vi "Main.vi"() -> ()   [LabVIEW 2017]
doc: "This template is for the Queued Message Handler design pattern.\n\nThe Event Handling Loop generates messages based on user interface actions.\n\nThe Message Handling Loop processes messages generated by the Event Handling Loop, or by other messages. The messages are string values, so new messages can be added easily to the Message Cases case structure in the Message Handling Loop. Each message cluster can also provide an optional value for Message Data, which is a variant that can be converted to whatever message-specific data is required."
uses:
  Entry Display Data.ctl
  support/Message Queue/Enqueue Message (Single).vi
  <vilib>/Utility/error.llb/Error Cluster From Error Code.vi
  <vilib>/ErrorRing/Error Ring.xnode
  support/Message Queue/Message Queue.lvlib
  support/User Event - Stop/User Event - Stop.lvlib
panel:
  in  "Start":bool
  in  "Air Dry":bool
  in  "Tire Shine Foam":bool
  in  "Spot Free Rinse":bool
  in  "Low Pressure Wax":bool
  in  "High Pressure Wash":bool
  in  "Pre-Soak":bool
  in  "Bug Remover":bool
  in  "Under Body Wash":bool
  out "Display <Replace Me>":string
  in  "Do Something Else <Replace Me>":bool
  in  "Do Something <Replace Me>":bool
  in  "Exit":bool
  # "These controls have associated \"Value Changed\" events configured in the Event Structure on the diagram.\n\nReplace them (and reconfigure the Event Structure) with the controls you need for your application."
  # "This template is for the Queued Message Handler design pattern.\n\nSee the block diagram for more information on how to use this template."
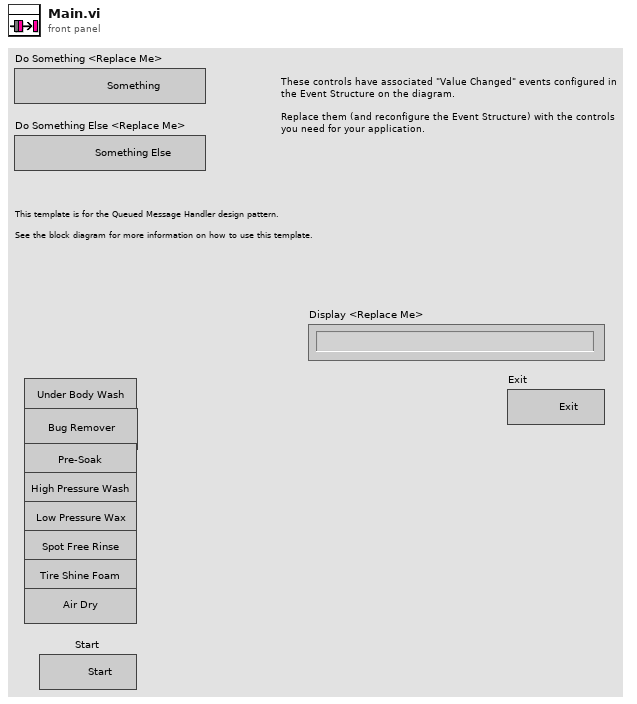
[diagram p1: front panel]
types:
  T1 = typedef "Entry Display Data.ctl" = cluster{"Under Body Wash":bool, "Bug Remover":bool, "Pre-soak":bool, " High Pressure Wash":bool, "Low Pressure  Wax":bool, "Spot Free Rinse":bool, " Tire Shine Foam":bool, " Air Dry":bool, "Vehicle Postion":bool}
  T2 = typedef "Message Queue.lvlib/All Message Queues.ctl" = cluster{"MHL":refnum<queue>, "Controller":refnum<queue>, "Display":refnum<queue>}
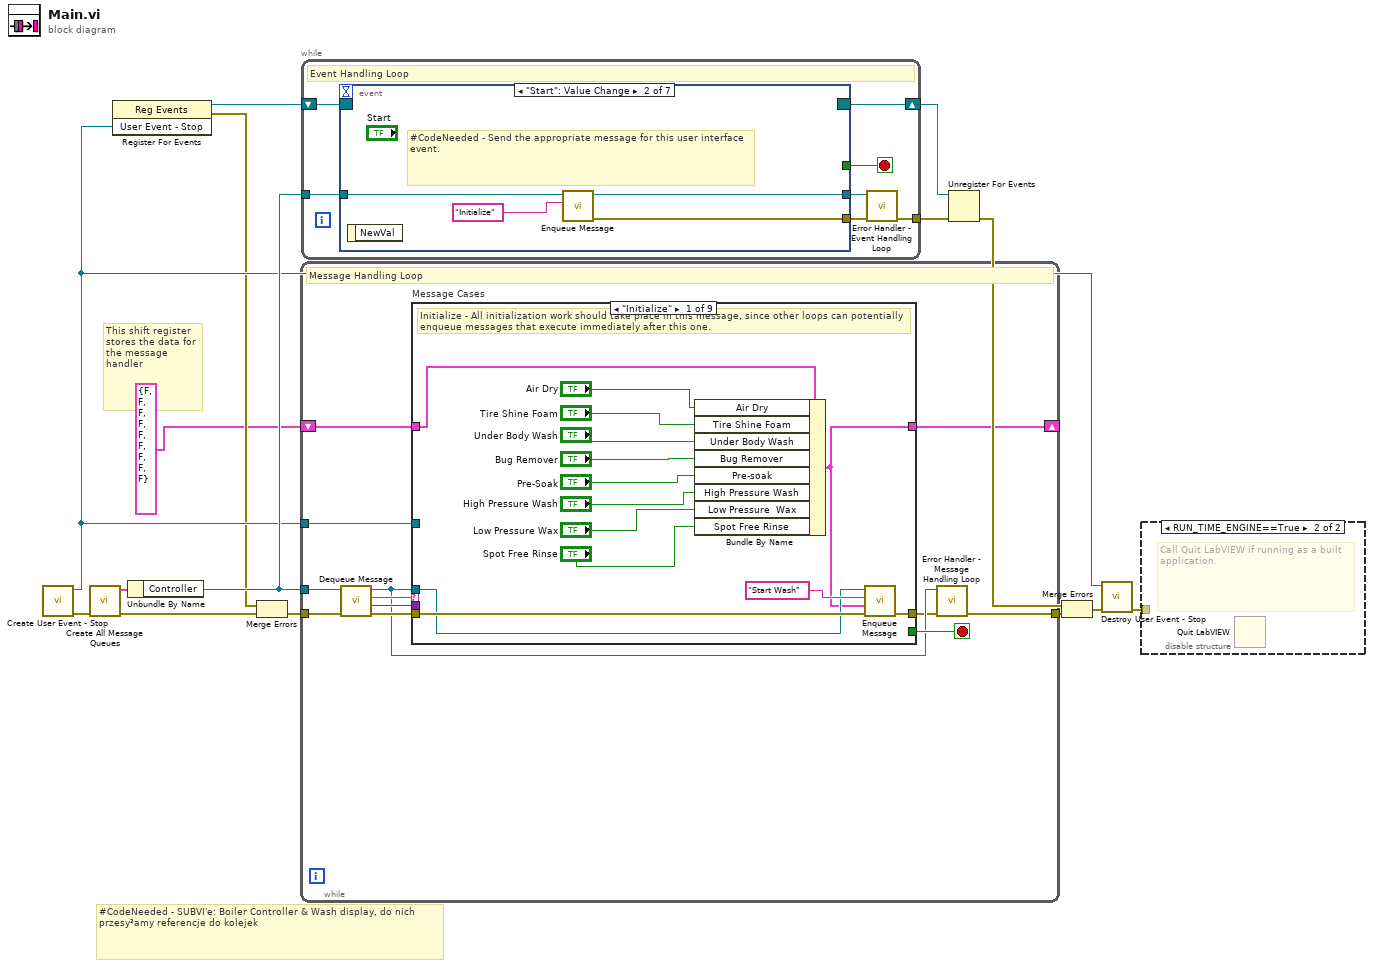
[diagram p0: block diagram]
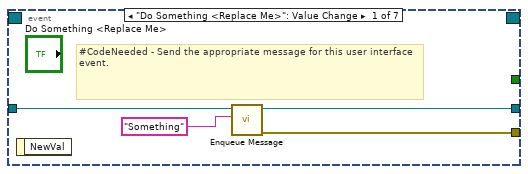
[diagram p3: hidden frame]
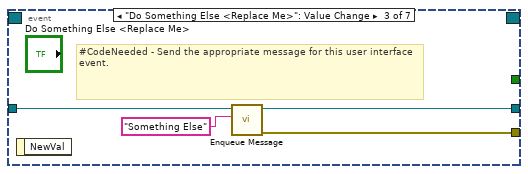
[diagram p4: hidden frame]
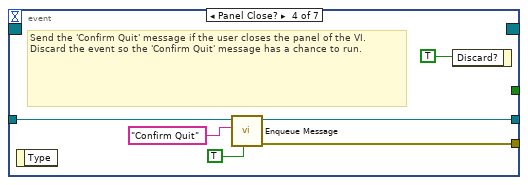
[diagram p5: hidden frame]
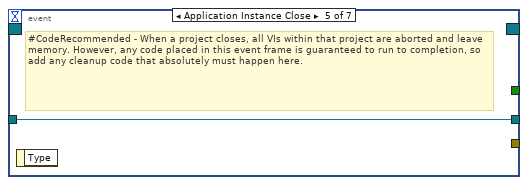
[diagram p6: hidden frame]
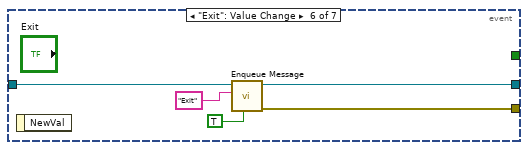
[diagram p7: hidden frame]
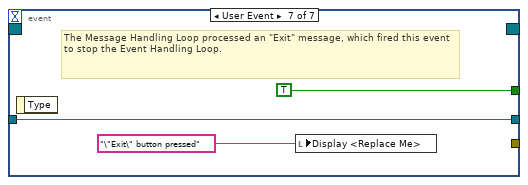
[diagram p8: hidden frame]
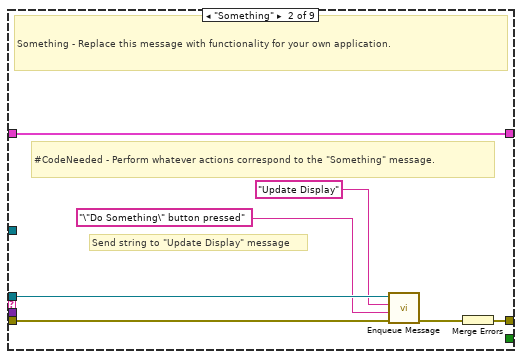
[diagram p9: hidden frame]
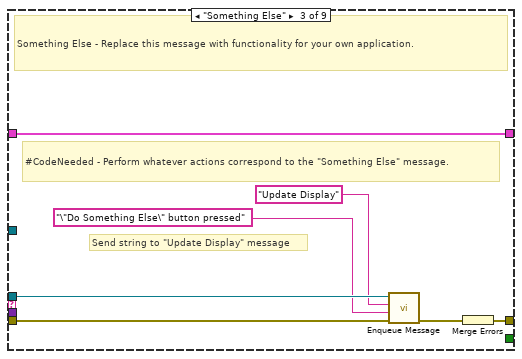
[diagram p10: hidden frame]
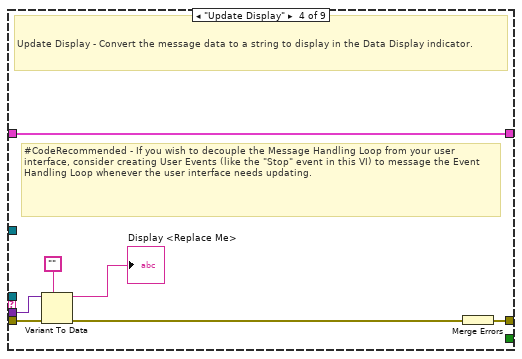
[diagram p11: hidden frame]
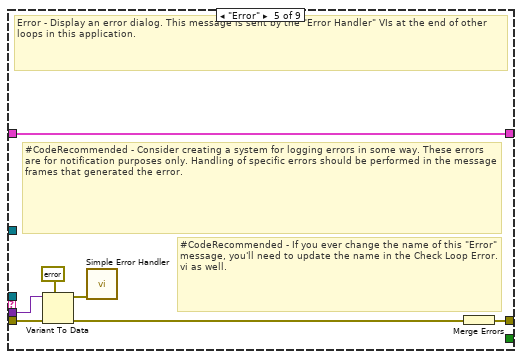
[diagram p12: hidden frame]
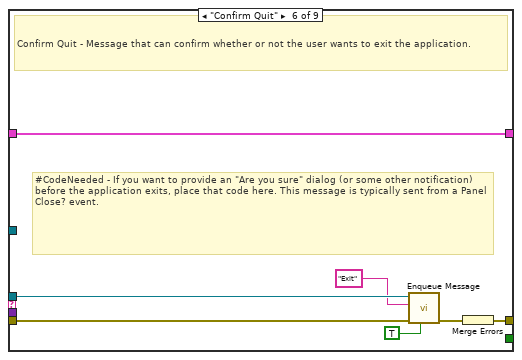
[diagram p13: hidden frame]
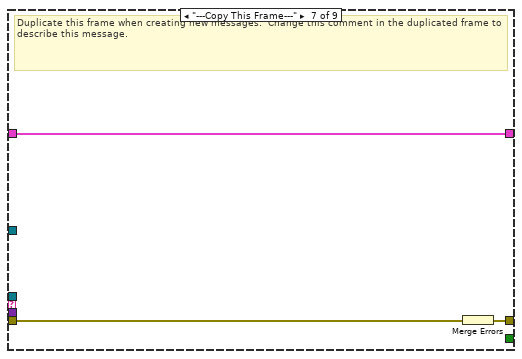
[diagram p14: hidden frame]
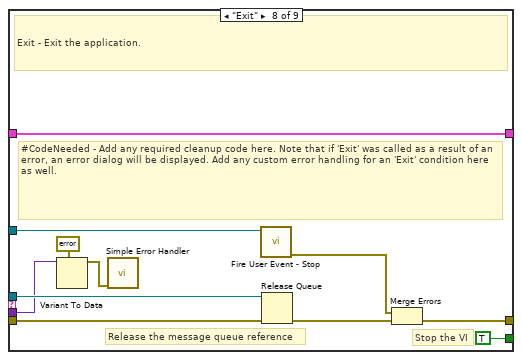
[diagram p15: hidden frame]
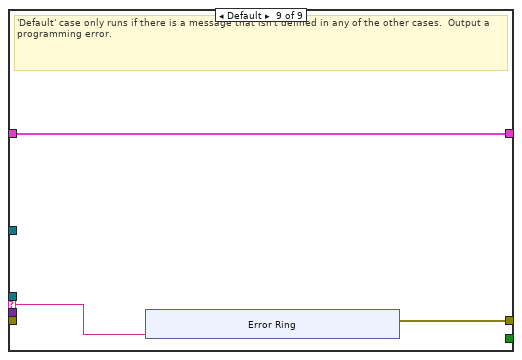
[diagram p16: hidden frame]
diagram:
  # "#CodeNeeded - SUBVI'e: Boiler Controller & Wash display, do nich przesy³amy referencje do kolejek"
  # "This shift register stores the data for the message handler"
  n1 = call "Create User Event - Stop.vi"() -> ("error out"=w11:errorcluster, "User Event - Stop"=w4:refnum<user-event>)  [unwired: 10 in]
  n2 = call "Create All Message Queues.vi"("error in (no error)"=w11) -> ("error out"=w15:errorcluster, "Message Queues out"=w14:T2)  [unwired: 9 in]
  n3 = register-events(w4) -> (reference out=w5:refnum<event-registration>, error out=w2:errorcluster)  [unwired: 2 in]
  n4 = Unbundle By Name(w14) -> ("Controller"=w12:refnum<queue>)
  n5 = Merge Errors(w2, w15) -> (w3:errorcluster)
  n6 = while {
    tunnel: w12 -> [w19]
    shift-right: [w26] -> _
    shift-left: T1 {"Under Body Wash"=FALSE, "Bug Remover"=FALSE, "Pre-soak"=FALSE, " High Pressure Wash"=FALSE, "Low Pressure  Wax"=FALSE, "Spot Free Rinse"=FALSE, " Tire Shine Foam"=FALSE, " Air Dry"=FALSE, "Vehicle Postion"=FALSE} ("Cluster") -> [w27]
    tunnel: w4 -> [w24]
    tunnel: w3 -> [w23]
    tunnel: [w17] -> w13
    stop <- w25 stop-if-true
    # "Message Handling Loop"
    n7 = call "Dequeue Message.vi"("error in (no error)"=w23, "Message Queue"=w19) -> ("error out"=w22:errorcluster, "Message Data"=w20:variant, "Message"=w21:string, "dup Message Queue"=w18:refnum<queue>)  [unwired: 6 in]
    n8 = case "Message Cases" shown="\"Initialize\"" w21 {
      selector: w21 -> [_ _ _ _ _ _ _ _ w91]
      tunnel: w18 -> [w38 w44 w51 _ _ w72 _ w90 _]
      tunnel: w22 -> [w40 w46 w53 w60 w69 w76 w79 w83 _]
      tunnel: [w41 w47 w54 w61 w63 w74 w77 w86 w92] -> w16
      tunnel: w27 -> [w29 w48 w55 w62 w68 w75 w78 w89 w93]
      tunnel: [w28 w48 w55 w62 w68 w75 w78 w89 w93] -> w26
      tunnel: [_ _ _ _ _ _ _ TRUE _] -> w25
      tunnel: w20 -> [_ _ _ w59 w67 _ _ w80 _]
      tunnel: w24 -> [_ _ _ _ _ _ _ w85 _]
      frame "Initialize" {
        # "Initialize - All initialization work should take place in this message, since other loops can potentially enqueue messages that execute immediately after this one."
        n9 = Bundle By Name(cluster=w29, "Air Dry"="Air Dry", "Tire Shine Foam"="Tire Shine Foam", "Under Body Wash"="Under Body Wash", "Bug Remover"="Bug Remover", "Pre-soak"="Pre-Soak", "High Pressure Wash"="High Pressure Wash", "Low Pressure  Wax"="Low Pressure Wax", "Spot Free Rinse"="Spot Free Rinse") -> (w28:T1)
        n10 = call-poly "Enqueue Message.vi"("error in (no error)"=w40, "Message Data"=w28, "Message"="Start Wash", "Message Queue"=w38) -> ("error out"=w41:errorcluster)  [unwired: 6 in, 1 out]
      }
      frame "Something" {
        # "Send string to \"Update Display\" message"
        # "#CodeNeeded - Perform whatever actions correspond to the \"Something\" message."
        # "Something - Replace this message with functionality for your own application."
        n11 = call-poly "Enqueue Message.vi"("error in (no error)"=w46, "Message Data"="\"Do Something\" button pressed" ("\"Do Something\" button pressed"), "Message"="Update Display", "Message Queue"=w44) -> ("error out"=w45:errorcluster)  [unwired: 6 in, 1 out]
        n12 = Merge Errors(w45) -> (w47:errorcluster)
      }
      frame "Something Else" {
        # "Send string to \"Update Display\" message"
        # "#CodeNeeded - Perform whatever actions correspond to the \"Something Else\" message."
        # "Something Else - Replace this message with functionality for your own application."
        n13 = call-poly "Enqueue Message.vi"("error in (no error)"=w53, "Message Data"="\"Do Something Else\" button pressed" ("\"Do Something Else\" button pressed"), "Message"="Update Display", "Message Queue"=w51) -> ("error out"=w52:errorcluster)  [unwired: 6 in, 1 out]
        n14 = Merge Errors(w52) -> (w54:errorcluster)
      }
      frame "Update Display" {
        # "#CodeRecommended - If you wish to decouple the Message Handling Loop from your user interface, consider creating User Events (like the \"Stop\" event in this VI) to message the Event Handling Loop whenever the user interface needs updating."
        # "Update Display - Convert the message data to a string to display in the Data Display indicator."
        n15 = Variant To Data(error in=w60, type="", Variant=w59) -> (data=→"Display <Replace Me>":string, error out=w57:errorcluster)
        n16 = Merge Errors(w57) -> (w61:errorcluster)
      }
      frame "Error" {
        # "#CodeRecommended - If you ever change the name of this \"Error\" message, you'll need to update the name in the Check Loop Error.vi as well."
        # "#CodeRecommended - Consider creating a system for logging errors in some way. These errors are for notification purposes only. Handling of specific errors should be performed in the message frames that generated the error."
        # "Error - Display an error dialog. This message is sent by the \"Error Handler\" VIs at the end of other loops in this application."
        n17 = Variant To Data(error in=w69, type=errorcluster {"status"=FALSE, "code"=0, "source"=""} ("error constant"), Variant=w67) -> (data=w65:errorcluster, error out=w64:errorcluster)
        n18 = call <vilib>:"Simple Error Handler.vi"("error in (no error)"=w65) -> ()  [unwired: 4 in, 5 out]
        n19 = Merge Errors(w64) -> (w63:errorcluster)
      }
      frame "Confirm Quit" {
        # "#CodeNeeded - If you want to provide an \"Are you sure\" dialog (or some other notification) before the application exits, place that code here. This message is typically sent from a Panel Close? event."
        # "Confirm Quit - Message that can confirm whether or not the user wants to exit the application."
        n20 = call-poly "Enqueue Message.vi"("Priority Message? (F)"=TRUE, "error in (no error)"=w76, "Message"="Exit", "Message Queue"=w72) -> ("error out"=w73:errorcluster)  [unwired: 6 in, 1 out]
        n21 = Merge Errors(w73) -> (w74:errorcluster)
      }
      frame "---Copy This Frame---" {
        # "Duplicate this frame when creating new messages.  Change this comment in the duplicated frame to describe this message."
        n22 = Merge Errors(w79) -> (w77:errorcluster)
      }
      frame "Exit" {
        # "Stop the VI"
        # "Release the message queue reference"
        # "#CodeNeeded - Add any required cleanup code here. Note that if 'Exit' was called as a result of an error, an error dialog will be displayed. Add any custom error handling for an 'Exit' condition here as well."
        # "Exit - Exit the application."
        n23 = Variant To Data(type=errorcluster {"status"=FALSE, "code"=0, "source"=""} ("error constant"), Variant=w80) -> (data=w81:errorcluster)  [unwired: 1 in, 1 out]
        n24 = call <vilib>:"Simple Error Handler.vi"("error in (no error)"=w81) -> ()  [unwired: 4 in, 5 out]
        n25 = call "Fire User Event - Stop.vi"("User Event - Stop"=w85) -> ("error out"=w84:errorcluster)  [unwired: 10 in]
        n26 = Release Queue(queue=w90, error in (no error)=w83) -> (error out=w87:errorcluster)  [unwired: 1 in, 2 out]
        n27 = Merge Errors(w84, w87) -> (w86:errorcluster)
      }
      frame Default {
        # "'Default' case only runs if there is a message that isn't defined in any of the other cases.  Output a programming error."
        n28 = xnode "Error Ring"("parameter 0"=w91) -> ("error out"=w92:errorcluster)
      }
    }
    n29 = call "Error Handler - Message Handling Loop.vi"("error in (no error)"=w16, "Message Queue"=w18) -> ("dup error in"=w17:errorcluster)  [unwired: 8 in, 1 out]
  }
  n30 = while {
    tunnel: w12 -> [w107]
    shift-right: [w105] -> w8
    shift-left: w5 -> [w106]
    tunnel: [w101] -> w6
    stop <- w103 stop-if-true
    # "Event Handling Loop"
    n31 = event shown="[1] \"Start\": Value Change" {
      selector: w106 -> [_ _ _ _ _ _ _]
      dyn-events: [_ _ _ _ _ _ _] -> w105
      timeout: _ -> [_ _ _ _ _ _ _]
      tunnel: [_ _ _ _ _ _ TRUE ("Discard?")] -> w103
      tunnel: w107 -> [w111 w115 w119 w124 w126 w131 w134]
      tunnel: [w108 w112 w116 w123 _ w130 _] -> w104
      tunnel: [w110 w114 w118 w122 w126 w129 w134] -> w102
      event "Do Something <Replace Me>": Value Change {
        # "#CodeNeeded - Send the appropriate message for this user interface event."
        n32 = event-data() -> ()  [unwired: 1 in, 1 out]
        n33 = call-poly "Enqueue Message.vi"("Message"="Something", "Message Queue"=w111) -> ("error out"=w108:errorcluster, "dup Message Queue"=w110:refnum<queue>)  [unwired: 8 in]
      }
      event "Start": Value Change {
        # "#CodeNeeded - Send the appropriate message for this user interface event."
        n34 = event-data() -> ()  [unwired: 1 in, 1 out]
        n35 = call-poly "Enqueue Message.vi"("Message"="Initialize", "Message Queue"=w115) -> ("error out"=w112:errorcluster, "dup Message Queue"=w114:refnum<queue>)  [unwired: 8 in]
      }
      event "Do Something Else <Replace Me>": Value Change {
        # "#CodeNeeded - Send the appropriate message for this user interface event."
        n36 = event-data() -> ()  [unwired: 1 in, 1 out]
        n37 = call-poly "Enqueue Message.vi"("Message"="Something Else", "Message Queue"=w119) -> ("error out"=w116:errorcluster, "dup Message Queue"=w118:refnum<queue>)  [unwired: 8 in]
      }
      event Panel Close? {
        # "Send the 'Confirm Quit' message if the user closes the panel of the VI. Discard the event so the 'Confirm Quit' message has a chance to run."
        n38 = event-data() -> ()  [unwired: 1 in, 1 out]
        n39 = call-poly "Enqueue Message.vi"("Priority Message? (F)"=TRUE, "Message"="Confirm Quit", "Message Queue"=w124) -> ("error out"=w123:errorcluster, "dup Message Queue"=w122:refnum<queue>)  [unwired: 7 in]
        n40 = event-data("Discard?"=TRUE) -> ()  [unwired: 1 in, 1 out]
      }
      event Application Instance Close {
        # "#CodeRecommended - When a project closes, all VIs within that project are aborted and leave memory. However, any code placed in this event frame is guaranteed to run to completion, so add any cleanup code that absolutely must happen here."
        n41 = event-data() -> ()  [unwired: 1 in, 1 out]
      }
      event "Exit": Value Change {
        n42 = event-data() -> ()  [unwired: 1 in, 1 out]
        n43 = call-poly "Enqueue Message.vi"("Priority Message? (F)"=TRUE, "Message"="Exit", "Message Queue"=w131) -> ("error out"=w130:errorcluster, "dup Message Queue"=w129:refnum<queue>)  [unwired: 7 in]
      }
      event User Event {
        # "The Message Handling Loop processed an \"Exit\" message, which fired this event to stop the Event Handling Loop."
        n44 = event-data() -> ()  [unwired: 1 in, 1 out]
        n45 = local write "Display <Replace Me>"("\"Exit\" button pressed" ("VI Stopped")) -> ()
      }
    }
    n46 = call "Error Handler - Event Handling Loop.vi"("error in (no error)"=w104, "Message Queue"=w102) -> ("dup error in"=w101:errorcluster)  [unwired: 8 in, 1 out]
  }
  n47 = Unregister For Events(event registration refnum=w8, error in=w6) -> (error out=w9:errorcluster)
  n48 = Merge Errors(w9, w13) -> (w10:errorcluster)
  n49 = call "Destroy User Event - Stop.vi"("error in (no error)"=w10, "User Event - Stop"=w4) -> ("error out"=w7:errorcluster)  [unwired: 9 in]
  n50 = disable-structure shown="RUN_TIME_ENGINE==True" {
    disable-tunnel: w7 -> [_ _]
    frame condition #0 (active) {
    }
    frame condition #1 {
      # "Call Quit LabVIEW if running as a built application."
      n51 = Quit LabVIEW() -> ()  [unwired: 1 in]
    }
  }
